vi "BuiltStageSetupCommands.vi"(0 "Y Speed (mms)":dbl, 1 "Stop X":dbl, 2 "Start X":dbl, 3 "Overshoot":dbl, 4 "X Encoder resolution":dbl, 5 "Stage Visa":refnum<visa-resource-name>, 6 "X Speed (mms)":dbl, 7 "X Pixels Count":i32, 8 "Scan Mode":enum16{"Raster Scan", "Serpentine Scan"}(ring), 9 "Start Y":dbl, 10 "Invert Axis":bool, 11 "Stop Y":dbl, 13 "Y Lines Count":i32) -> (14 "Scan Time":dbl, 15 "X resolution":dbl, 16 "Y Resolution":dbl, 17 "Commands array":string[](array[string]), 19 "Stage Setup Info":T1)   [LabVIEW 2018]
uses:
  Controls/StageInfo.ctl
  Program_Files/Labview2018/MAIN/instr.lib/ASI TG-1000/ASI TG-1000.lvlib
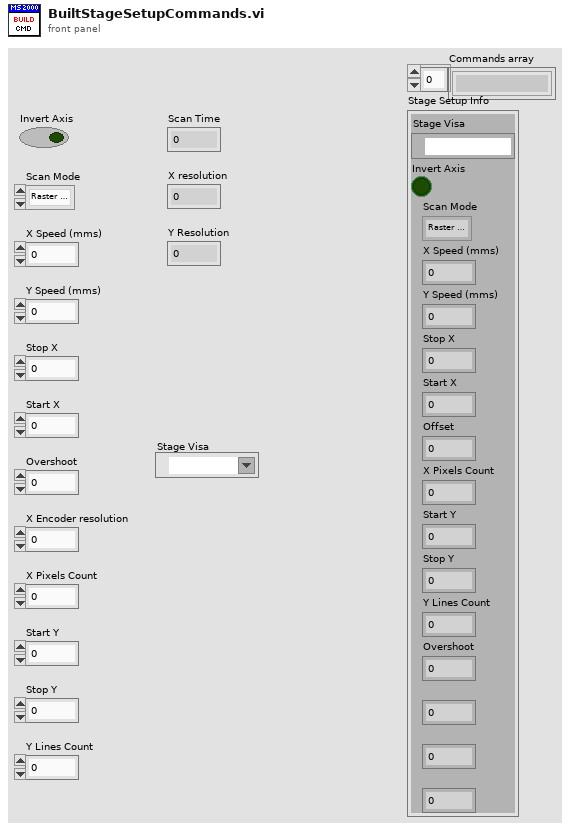
[diagram p1: front panel]
types:
  T1 = typedef "StageInfo.ctl" = cluster{"Stage Visa":refnum<visa-resource-name>, "Invert Axis":bool, "Scan Mode":enum16{"Raster Scan", "Serpentine Scan"}, "X Speed (mms)":dbl, "Y Speed (mms)":dbl, "Stop X":dbl, "Start X":dbl, "Offset":dbl, "X Pixels Count":i32, "Start Y":dbl, "Stop Y":dbl, "Y Lines Count":i32, "Overshoot":dbl, "Scan Time":dbl, "X Resolution":dbl, "Y Resolution":dbl}
  T2 = cluster{"Stage Visa":refnum<visa-resource-name>, "Invert Axis":bool, "Scan Mode":enum16{"Raster Scan", "Serpentine Scan"}, "X Speed (mms)":dbl, "Y Speed (mms)":dbl, "Stop X":dbl, "Start X":dbl, "y":dbl, "X Pixels Count":i32, "Start Y":dbl, "Stop Y":dbl, "Y Lines Count":i32, "Overshoot":dbl, dbl, dbl, dbl}
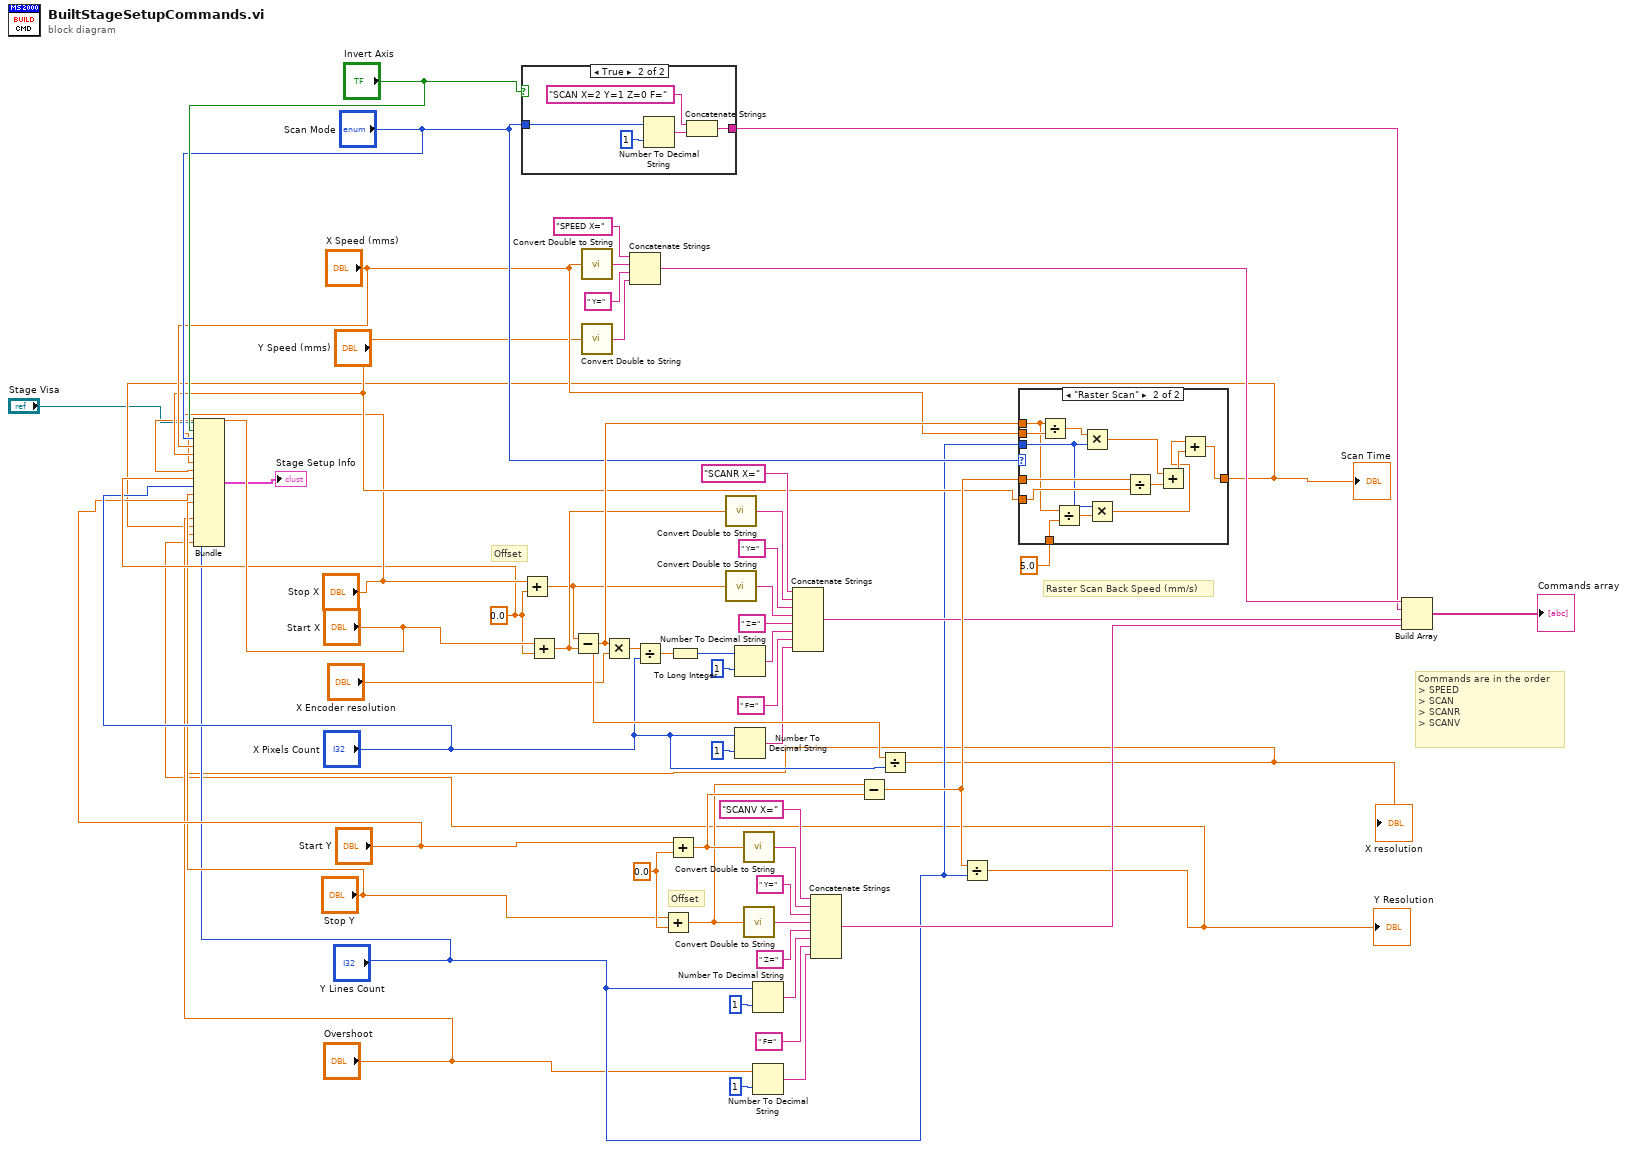
[diagram p0: block diagram]
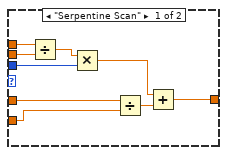
[diagram p2: hidden frame]
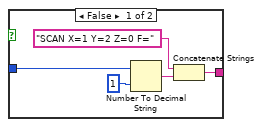
[diagram p3: hidden frame]
diagram:
  w48 = 0.0 ("y")
  w11 = 0.0 ("y")
  # "Commands are in the order\n> SPEED\n> SCAN \n> SCANR\n> SCANV"
  # "Raster Scan Back Speed (mm/s)"
  # "Offset"
  # "Offset"
  n1 = case shown="True" "Invert Axis" {
    tunnel: "Scan Mode" -> [w61 w65]
    tunnel: [w59 w64] -> w21
    frame False {
      n2 = Number To Decimal String(number=w61, width (-)=i16 1) -> (decimal integer string=w62:string)
      n3 = Concatenate Strings("SCAN X=1 Y=2 Z=0 F=" ("string"), w62) -> (w59:string)
    }
    frame True {
      n4 = Number To Decimal String(number=w65, width (-)=i16 1) -> (decimal integer string=w68:string)
      n5 = Concatenate Strings("SCAN X=2 Y=1 Z=0 F=" ("string"), w68) -> (w64:string)
    }
  }
  n6 = Add(x="Stop X", y=w11) -> (x+y=w33:dbl)
  n7 = Add(x="Start X", y=w11) -> (x+y=w34:dbl)
  n8 = Subtract(x=w33, y=w34) -> (x-y=w56:dbl)
  n9 = call "Convert Double to String.vi"("Value"="X Speed (mms)") -> ("String"=w27:string)
  n10 = call "Convert Double to String.vi"("Value"="Y Speed (mms)") -> ("String"=w28:string)
  n11 = Multiply(x=w56, y="X Encoder resolution") -> (x*y=w35:dbl)
  n12 = Concatenate Strings("SPEED X=" ("string"), w27, " Y=" ("string"), w28) -> (w22:string)
  n13 = Divide(x=w35, y="X Pixels Count") -> (x/y=w36:dbl)
  n14 = Add(x="Stop Y", y=w48) -> (x+y=w54:dbl)
  n15 = Add(x="Start Y", y=w48) -> (x+y=w55:dbl)
  n16 = To Long Integer(number=w36) -> (32bit integer=w38:i32)
  n17 = call "Convert Double to String.vi"("Value"=w34) -> ("String"=w26:string)
  n18 = call "Convert Double to String.vi"("Value"=w33) -> ("String"=w30:string)
  n19 = Number To Decimal String(number=w38, width (-)=i16 1) -> (decimal integer string=w39:string)
  n20 = Number To Decimal String(number="X Pixels Count", width (-)=i16 1) -> (decimal integer string=w42:string)
  n21 = call "Convert Double to String.vi"("Value"=w55) -> ("String"=w44:string)
  n22 = call "Convert Double to String.vi"("Value"=w54) -> ("String"=w46:string)
  n23 = Number To Decimal String(number="Y Lines Count", width (-)=i16 1) -> (decimal integer string=w50:string)
  n24 = Number To Decimal String(number="Overshoot", width (-)=i16 1) -> (decimal integer string=w53:string)
  n25 = Concatenate Strings("SCANR X=" ("string"), w26, " Y=" ("string"), w30, " Z=" ("string"), w39, " F=" ("string"), w42) -> (w20:string)
  n26 = Concatenate Strings("SCANV X=" ("string"), w44, " Y=" ("string"), w46, " Z=" ("string"), w50, " F=" ("string"), w53) -> (w19:string)
  n27 = Subtract(x=w54, y=w55) -> (x-y=w57:dbl)
  n28 = Divide(x=w56, y="X Pixels Count") -> (x/y=w4:dbl)
  "X resolution" <- w4
  n29 = Divide(x=w57, y="Y Lines Count") -> (x/y=w3:dbl)
  "Y Resolution" <- w3
  n30 = case shown="\"Raster Scan\"" "Scan Mode" {
    tunnel: "X Speed (mms)" -> [w77 w90]
    tunnel: w56 -> [w76 w79]
    tunnel: "Y Lines Count" -> [w75 w82]
    tunnel: w57 -> [w71 w86]
    tunnel: "Y Speed (mms)" -> [w70 w85]
    tunnel: [w69 w84] -> w5
    tunnel: 5.0 -> [_ w78]
    frame "Serpentine Scan" {
      n31 = Divide(x=w76, y=w77) -> (x/y=w74:dbl)
      n32 = Multiply(x=w74, y=w75) -> (x*y=w73:dbl)
      n33 = Divide(x=w71, y=w70) -> (x/y=w72:dbl)
      n34 = Add(x=w73, y=w72) -> (x+y=w69:dbl)
    }
    frame "Raster Scan" {
      n35 = Divide(x=w79, y=w90) -> (x/y=w89:dbl)
      n36 = Divide(x=w79, y=w78) -> (x/y=w80:dbl)
      n37 = Multiply(x=w89, y=w82) -> (x*y=w88:dbl)
      n38 = Multiply(x=w82, y=w80) -> (x*y=w81:dbl)
      n39 = Divide(x=w86, y=w85) -> (x/y=w87:dbl)
      n40 = Add(x=w88, y=w87) -> (x+y=w83:dbl)
      n41 = Add(x=w81, y=w83) -> (x+y=w84:dbl)
    }
  }
  "Scan Time" <- w5
  n42 = Bundle("Stage Visa"="Stage Visa", "Invert Axis"="Invert Axis", "Scan Mode"="Scan Mode", "X Speed (mms)"="X Speed (mms)", "Y Speed (mms)"="Y Speed (mms)", "Stop X"="Stop X", "Start X"="Start X", "y"=w11, "X Pixels Count"="X Pixels Count", "Start Y"="Start Y", "Stop Y"="Stop Y", "Y Lines Count"="Y Lines Count", "Overshoot"="Overshoot", w5, w4, w3) -> (→"Stage Setup Info":T2)  [unwired: 1 in]
  n43 = Build Array(w22, w21, w20, w19) -> (→"Commands array":string[])
